vi "minicryo_T-control_He3.vi"(0 "Mini Set":dbl, 5 "Ramp Mode":bool, 7 "Rate  [K/min]":dbl=0.1, 9 "VISA resource name out":refnum<visa-resource-name>="COM4", 11 "Set Main Temp [K]":dbl=1.5) -> ()   [LabVIEW 2013]
panel:
  in  "Heater":bool
  out "String":string="+023.261E+0;+022.689E+0\n"
  in  "Auto PID":bool=TRUE
  out "D1":string="0"
  out "I1":string="40"
  out "P1":string="120"
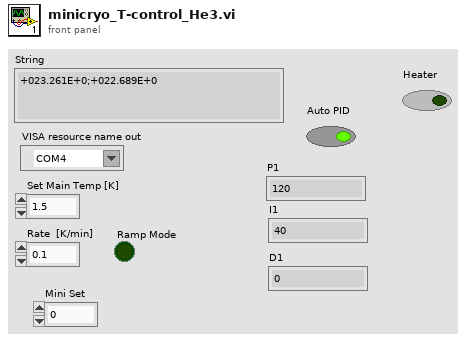
[diagram p1: front panel]
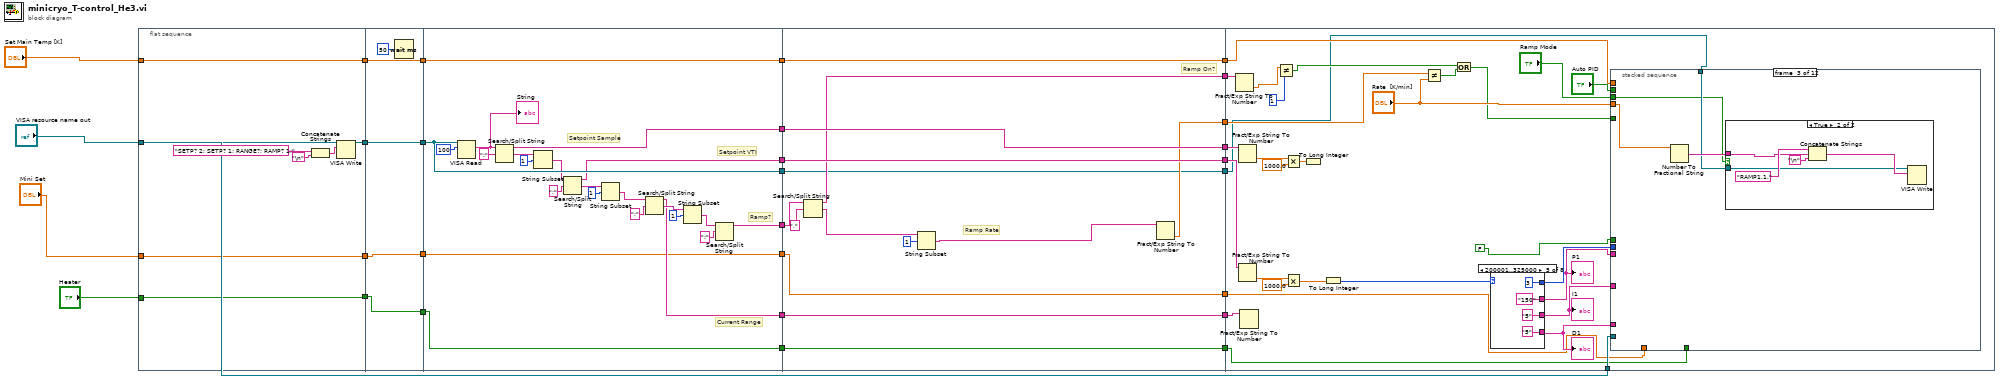
[diagram p0: block diagram]
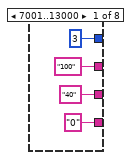
[diagram p2: hidden frame]
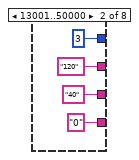
[diagram p3: hidden frame]
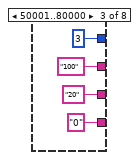
[diagram p4: hidden frame]
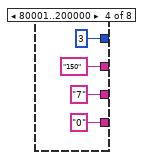
[diagram p5: hidden frame]
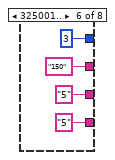
[diagram p6: hidden frame]
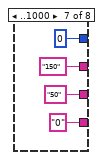
[diagram p7: hidden frame]
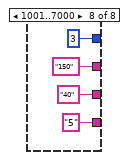
[diagram p8: hidden frame]
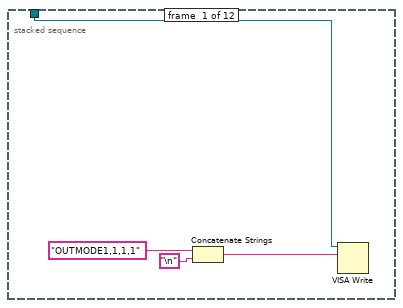
[diagram p9: hidden frame]
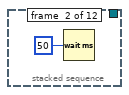
[diagram p10: hidden frame]
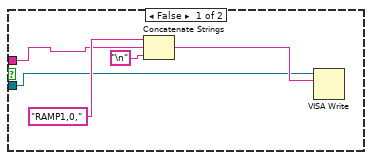
[diagram p11: hidden frame]
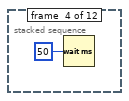
[diagram p12: hidden frame]
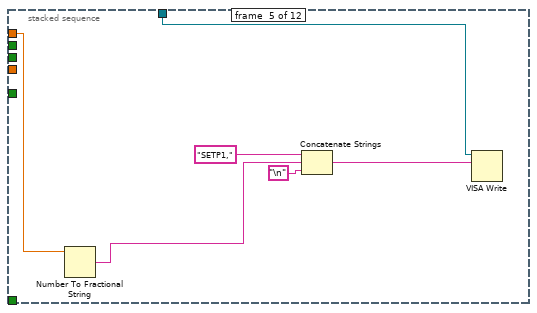
[diagram p13: hidden frame]
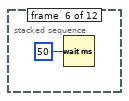
[diagram p14: hidden frame]
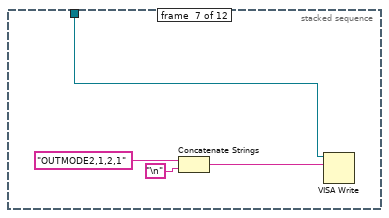
[diagram p15: hidden frame]
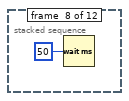
[diagram p16: hidden frame]
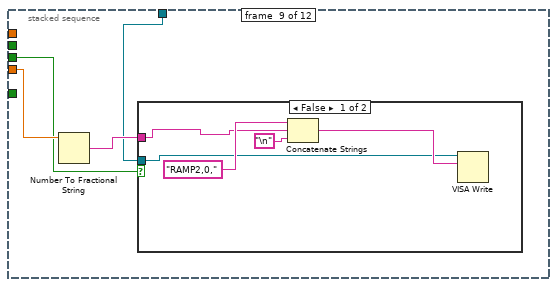
[diagram p17: hidden frame]
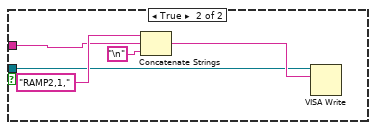
[diagram p18: hidden frame]
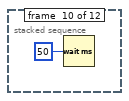
[diagram p19: hidden frame]
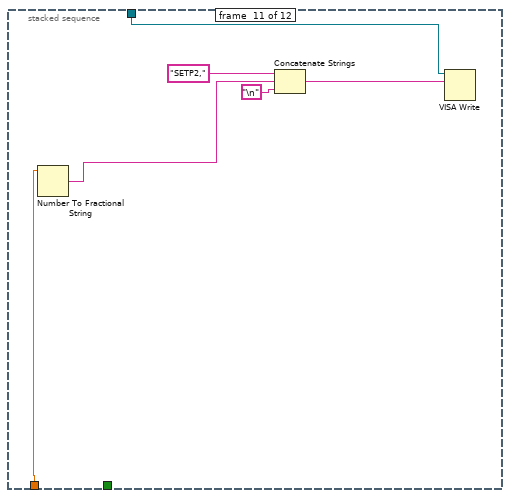
[diagram p20: hidden frame]
diagram:
  n1 = flat-sequence {
    tunnel: "VISA resource name out" -> [w33]
    tunnel: "Set Main Temp [K]" -> [w37]
    tunnel: [w37] -> w22
    tunnel: [w32] -> w21
    tunnel: [w31] -> w10
    tunnel: "Heater" -> [w31]
    tunnel: [w30] -> w5
    tunnel: "Mini Set" -> [w30]
    tunnel: [w42] -> w24
    tunnel: [w41] -> w23
    tunnel: w22 -> [w42]
    tunnel: w21 -> [w41]
    tunnel: w10 -> [w39]
    tunnel: [w39] -> w8
    tunnel: w5 -> [w38]
    tunnel: [w38] -> w2
    tunnel: [w65] -> w26
    tunnel: [w63] -> w25
    tunnel: w24 -> [w65]
    tunnel: w23 -> [w63]
    tunnel: [w59] -> w20
    tunnel: [w53] -> w19
    tunnel: [w47] -> w15
    tunnel: [w45] -> w14
    tunnel: w8 -> [w44]
    tunnel: [w44] -> w7
    tunnel: [w43] -> w3
    tunnel: w2 -> [w43]
    tunnel: [w79] -> w27
    tunnel: [w78] -> w18
    tunnel: [w77] -> w17
    tunnel: [w76] -> w16
    tunnel: w26 -> [w79]
    tunnel: w25 -> [w68]
    tunnel: w20 -> [w77]
    tunnel: w19 -> [w78]
    tunnel: w15 -> [w76]
    tunnel: w14 -> [w75]
    tunnel: [w73] -> w13
    tunnel: [w69] -> w12
    tunnel: [w68] -> w11
    tunnel: w7 -> [w67]
    tunnel: [w67] -> w6
    tunnel: w3 -> [w66]
    tunnel: [w66] -> w1
    tunnel: "VISA resource name out" -> [w99]
    tunnel: w27 -> [w94]
    tunnel: w18 -> [w98]
    tunnel: w17 -> [w96]
    tunnel: w16 -> [w93]
    tunnel: w13 -> [w91]
    tunnel: w12 -> [w87]
    tunnel: w11 -> [w83]
    tunnel: w6 -> [w82]
    tunnel: w1 -> [w81]
    frame #0 {
      n2 = Concatenate Strings("SETP? 2; SETP? 1; RANGE?; RAMP? 1;" ("write buffer"), "\n") -> (w34:string)
      n3 = VISA Write(VISA resource name=w33, write buffer=w34) -> (VISA resource name out=w32:refnum<visa-resource-name>)  [unwired: 1 in, 2 out]
    }
    frame #1 {
      n4 = Wait (ms)(milliseconds to wait=50) -> ()  [unwired: 1 out]
    }
    frame #2 {
      # "Ramp?"
      # "Current Range"
      # "Setpoint VTI"
      # "Setpoint Sample"
      n5 = VISA Read(VISA resource name=w63, byte count=u32 100) -> (read buffer=w58:string)  [unwired: 1 in, 3 out]
      "String" <- w58
      n6 = Search/Split String(string=w58, search string/char (-)=";") -> (substring before match=w59:string, match + rest of string=w61:string)  [unwired: 1 in, 1 out]
      n7 = String Subset(string=w61, offset (0)=u32 1 ("byte count")) -> (substring=w54:string)  [unwired: 1 in]
      n8 = Search/Split String(string=w54, search string/char (-)=";") -> (substring before match=w53:string, match + rest of string=w57:string)  [unwired: 1 in, 1 out]
      n9 = String Subset(string=w57, offset (0)=u32 1 ("byte count")) -> (substring=w48:string)  [unwired: 1 in]
      n10 = Search/Split String(string=w48, search string/char (-)=";") -> (substring before match=w47:string, match + rest of string=w52:string)  [unwired: 1 in, 1 out]
      n11 = String Subset(string=w52, offset (0)=u32 1 ("byte count")) -> (substring=w46:string)  [unwired: 1 in]
      n12 = Search/Split String(string=w46, search string/char (-)=";") -> (substring before match=w45:string)  [unwired: 1 in, 2 out]
    }
    frame #3 {
      # "Ramp Rate"
      # "Ramp On?"
      n13 = Search/Split String(string=w75, search string/char (-)=",") -> (substring before match=w73:string, match + rest of string=w71:string)  [unwired: 1 in, 1 out]
      n14 = String Subset(string=w71, offset (0)=u32 1 ("byte count")) -> (substring=w70:string)  [unwired: 1 in]
      n15 = Fract/Exp String To Number(string=w70) -> (number=w69:dbl)  [unwired: 3 in, 1 out]
    }
    frame #4 {
      n16 = Fract/Exp String To Number(string=w91) -> (number=w90:dbl)  [unwired: 3 in, 1 out]
      n17 = Fract/Exp String To Number(string=w96) -> (number=w95:dbl)  [unwired: 3 in, 1 out]
      n18 = Fract/Exp String To Number(string=w98) -> (number=w97:dbl)  [unwired: 3 in, 1 out]
      n19 = Fract/Exp String To Number(string=w93) -> ()  [unwired: 3 in, 2 out]
      n20 = Not Equal?(x=w90, y=1) -> (x != y?=w85:bool)
      n21 = Multiply(x=w95, y=1000.0) -> (x*y=w108:dbl)
      n22 = Multiply(x=w97, y=1000.0) -> (x*y=w105:dbl)
      n23 = To Long Integer(number=w108) -> ()  [unwired: 1 out]
      n24 = To Long Integer(number=w105) -> (32bit integer=w104:i32)
      n25 = Not Equal?(x=w87, y="Rate  [K/min]") -> (x != y?=w86:bool)
      n26 = Or(x=w85, y=w86) -> (x .or. y?=w84:bool)
      n27 = case shown="200001..325000" w104 {
        tunnel: [3 3 3 3 3 3 0 3] -> w92
        tunnel: ["100" "120" "100" "150" "150" "150" "150" "150"] -> w103
        tunnel: ["40" "40" "20" "7" "5" "5" "50" "40"] -> w102
        tunnel: ["0" "0" "0" "0" "5" "5" "0" "5"] -> w101
        frame 7001..13000 {
        }
        frame 13001..50000 {
        }
        frame 50001..80000 {
        }
        frame 80001..200000 {
        }
        frame 200001..325000 {
        }
        frame 325001.. {
        }
        frame ..1000 {
        }
        frame 1001..7000 {
        }
      }
      "P1" <- w103
      "I1" <- w102
      "D1" <- w101
      n28 = stacked-sequence {
        tunnel: w99 -> [_ _ _ _ _ _ _ _ _ _ _ _]
        tunnel: "Rate  [K/min]" -> [_ _ w148 _ _ _ _ _ w175 _ _ _]
        tunnel: "Ramp Mode" -> [_ _ w147 _ _ _ _ _ w174 _ _ _]
        tunnel: w94 -> [_ _ _ _ w162 _ _ _ _ _ _ _]
        tunnel: w92 -> [_ _ _ _ _ _ _ _ _ _ _ _]
        tunnel: w103 -> [_ _ _ _ _ _ _ _ _ _ _ _]
        tunnel: w102 -> [_ _ _ _ _ _ _ _ _ _ _ _]
        tunnel: w101 -> [_ _ _ _ _ _ _ _ _ _ _ _]
        tunnel: "Auto PID" -> [_ _ _ _ _ _ _ _ _ _ _ _]
        tunnel: FALSE -> [_ _ _ _ _ _ _ _ _ _ _ _]
        tunnel: w84 -> [_ _ _ _ _ _ _ _ _ _ _ _]
        tunnel: w83 -> [w142 _ w149 _ w163 _ w169 _ w176 _ w189 _]
        tunnel: w82 -> [_ _ _ _ _ _ _ _ _ _ _ _]
        tunnel: w81 -> [_ _ _ _ _ _ _ _ _ _ w190 _]
        frame #0 {
          n29 = Concatenate Strings("OUTMODE1,1,1,1" ("write buffer"), "\n") -> (w143:string)
          n30 = VISA Write(VISA resource name=w142, write buffer=w143) -> ()  [unwired: 1 in, 3 out]
        }
        frame #1 {
          n31 = Wait (ms)(milliseconds to wait=u32 50) -> ()  [unwired: 1 out]
        }
        frame #2 {
          n32 = Number To Fractional String(number=w148) -> (F-format string=w150:string)  [unwired: 3 in]
          n33 = case shown="True" w147 {
            tunnel: w150 -> [w152 w157]
            tunnel: w149 -> [w151 w156]
            frame False {
              n34 = Concatenate Strings("RAMP1,0," ("write buffer"), w152, "\n") -> (w154:string)
              n35 = VISA Write(VISA resource name=w151, write buffer=w154) -> ()  [unwired: 1 in, 3 out]
            }
            frame True {
              n36 = Concatenate Strings("RAMP1,1," ("write buffer"), w157, "\n") -> (w159:string)
              n37 = VISA Write(VISA resource name=w156, write buffer=w159) -> ()  [unwired: 1 in, 3 out]
            }
          }
        }
        frame #3 {
          n38 = Wait (ms)(milliseconds to wait=u32 50) -> ()  [unwired: 1 out]
        }
        frame #4 {
          n39 = Number To Fractional String(number=w162) -> (F-format string=w164:string)  [unwired: 3 in]
          n40 = Concatenate Strings("SETP1," ("write buffer"), w164, "\n") -> (w166:string)
          n41 = VISA Write(VISA resource name=w163, write buffer=w166) -> ()  [unwired: 1 in, 3 out]
        }
        frame #5 {
          n42 = Wait (ms)(milliseconds to wait=u32 50) -> ()  [unwired: 1 out]
        }
        frame #6 {
          n43 = Concatenate Strings("OUTMODE2,1,2,1" ("write buffer"), "\n") -> (w170:string)
          n44 = VISA Write(VISA resource name=w169, write buffer=w170) -> ()  [unwired: 1 in, 3 out]
        }
        frame #7 {
          n45 = Wait (ms)(milliseconds to wait=u32 50) -> ()  [unwired: 1 out]
        }
        frame #8 {
          n46 = Number To Fractional String(number=w175) -> (F-format string=w177:string)  [unwired: 3 in]
          n47 = case shown="False" w174 {
            tunnel: w177 -> [w179 w184]
            tunnel: w176 -> [w178 w183]
            frame False {
              n48 = Concatenate Strings("RAMP2,0," ("write buffer"), w179, "\n") -> (w181:string)
              n49 = VISA Write(VISA resource name=w178, write buffer=w181) -> ()  [unwired: 1 in, 3 out]
            }
            frame True {
              n50 = Concatenate Strings("RAMP2,1," ("write buffer"), w184, "\n") -> (w186:string)
              n51 = VISA Write(VISA resource name=w183, write buffer=w186) -> ()  [unwired: 1 in, 3 out]
            }
          }
        }
        frame #9 {
          n52 = Wait (ms)(milliseconds to wait=u32 50) -> ()  [unwired: 1 out]
        }
        frame #10 {
          n53 = Number To Fractional String(number=w190) -> (F-format string=w191:string)  [unwired: 3 in]
          n54 = Concatenate Strings("SETP2," ("write buffer"), w191, "\n") -> (w193:string)
          n55 = VISA Write(VISA resource name=w189, write buffer=w193) -> ()  [unwired: 1 in, 3 out]
        }
        frame #11 {
          n56 = Wait (ms)(milliseconds to wait=u32 50) -> ()  [unwired: 1 out]
        }
      }
    }
  }
